vi "SetResolution.vi"(8 "error in (no error)":errorcluster, 10 "Resolution":u8 format="%.0x", 11 "CameraTesting in":refnum<class "CameraTesting.lvclass">) -> (0 "error out":errorcluster, 3 "CameraTesting out":refnum<class "CameraTesting.lvclass">)   [LabVIEW 2020, in "CameraTesting.lvlib" / "CameraTesting.lvclass"]
uses:
  CameraTesting.lvclass
  CameraTesting.lvclass/CameraTesting.ctl
  Camera/ICamera/ICamera/ICamera.lvclass
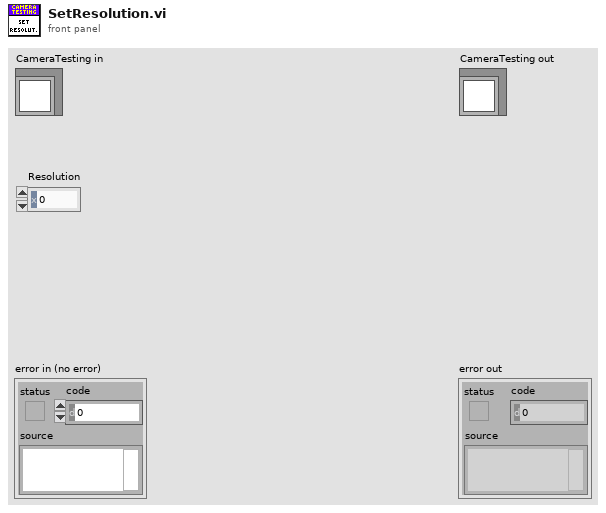
[diagram p1: front panel]
types:
  T1 = typedef "ICameraTesting.lvlib/ICameraTesting.lvclass/StatusUpdated.ctl" = refnum<user-event>
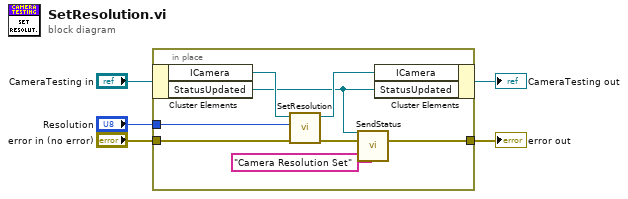
[diagram p0: block diagram]
diagram:
  n1 = in-place {
    in-place-border: "Resolution" -> [w13]
    in-place-border: "error in (no error)" -> [w12]
    in-place-border: [w7] -> w3
    n2 = in-place-cluster #1("CameraTesting in") -> ("ICamera"=w11:refnum<class "ICamera.lvclass">, "StatusUpdated"=w6:T1)
    n3 = call-dynamic "SetResolution.vi"("error in (no error)"=w12, "Resolution (hex code)"=w13, "ICamera in"=w11) -> ("error out"=w8:errorcluster, "ICamera out"=w10:refnum<class "ICamera.lvclass">)  [unwired: 7 in]
    n4 = call "SendStatus.vi"("StatusUsrEvn"=w6, "error in"=w8, "Text"="Camera Resolution Set") -> ("error out"=w7:errorcluster)  [unwired: 24 in]
    n5 = in-place-cluster #1("ICamera"=w10, "StatusUpdated"=w6) -> (→"CameraTesting out":refnum<class "CameraTesting.lvclass">)
  }
  "error out" <- w3
